vi "Get camera from name.vi"(0 "Red ref":refnum<k24>, 5 "Green ref":refnum<k24>, 7 "Blue ref":refnum<k24>, 9 "Camera":u16(ring) items=["Red", "Green", "Blue"], 11 "Error In":errorcluster) -> (4 "Camera reference out":refnum<k24>, 15 "Error Out":errorcluster)   [LabVIEW 2017]
uses:
  C:/Program Files/National Instruments/LabVIEW 2017/instr.lib/IDS/ueye.NET/uEyeDotNet.dll
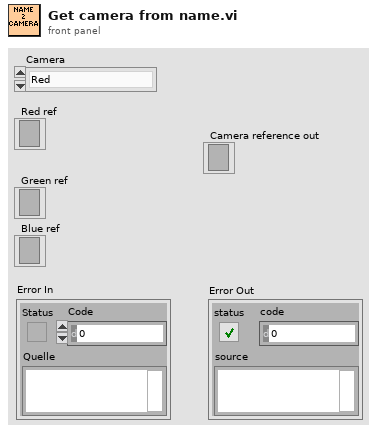
[diagram p1: front panel]
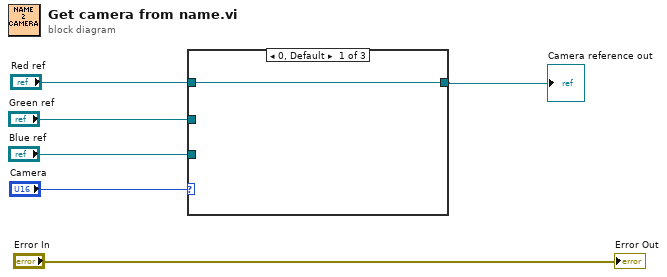
[diagram p0: block diagram]
diagram:
  n1 = case shown="0, Default" "Camera" {
    tunnel: "Blue ref" -> [_ _ w9]
    tunnel: "Green ref" -> [_ w8 _]
    tunnel: "Red ref" -> [w7 _ _]
    tunnel: [w7 w8 w9] -> w1
    frame 0, Default {
    }
    frame 1 {
    }
    frame 2 {
    }
  }
  "Camera reference out" <- w1
  "Error Out" <- "Error In"
